vi "dumps.vi"(8 "error in (no error)":errorcluster, 9 "remove comments? (F)":bool, 10 "sections":T1[](array[typedef]), 11 "path in":path) -> (0 "error out":errorcluster, 3 "path out":path)   [LabVIEW 2017, in "toml.lvlib"]
uses:
  toml.lvlib
  fg_section.ctl
  fg_row.ctl
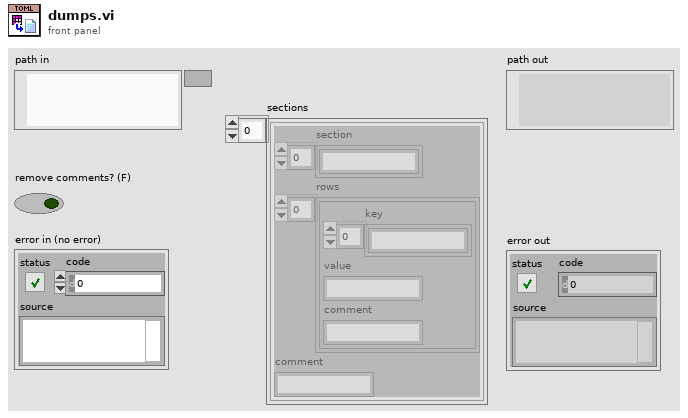
[diagram p1: front panel]
types:
  T1 = typedef "toml.lvlib/fg_section.ctl" = cluster{"section":string[], "rows":T2[], "comment":string}
  T2 = typedef "toml.lvlib/fg_row.ctl" = cluster{"key":string[], "value":string, "comment":string}
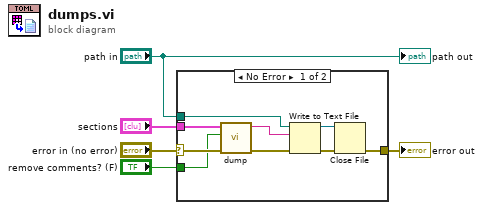
[diagram p0: block diagram]
diagram:
  n1 = case shown="No Error" "error in (no error)" {
    selector: "error in (no error)" -> [w14 w15]
    tunnel: "sections" -> [w12 _]
    tunnel: "remove comments? (F)" -> [w11 _]
    tunnel: [w9 w15] -> w2
    tunnel: "path in" -> [w6 _]
    frame No Error {
      n2 = call "dump.vi"("error in (no error)"=w14, "remove comments? (F)"=w11, "sections"=w12) -> ("error out"=w13:errorcluster, "toml"=w7:string)  [unwired: 7 in]
      n3 = Write to Text File(file (use dialog)=w6, text=w7, error in=w13) -> (refnum out=w8:refnum<file>, error out=w10:errorcluster)  [unwired: 1 in, 1 out]
      n4 = Close File(refnum=w8, error in=w10) -> (error out=w9:errorcluster)  [unwired: 1 out]
    }
    frame Error {
    }
  }
  "error out" <- w2
  "path out" <- "path in"
